vi "IsOpenInterface.vi"(10 "interface handle":i64, 11 "error in (no error)":errorcluster) -> (2 "return type":i8, 3 "error out":errorcluster)   [LabVIEW 2016]
uses:
  MVSDKmd.dll
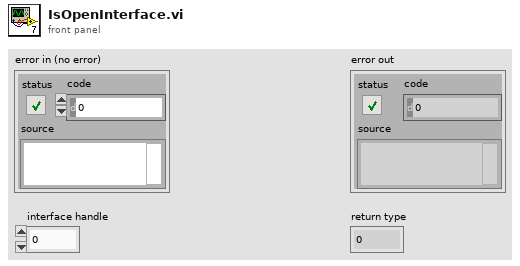
[diagram p1: front panel]
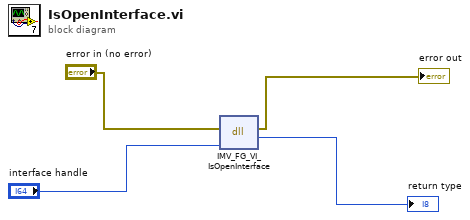
[diagram p0: block diagram]
diagram:
  n1 = dll-call lib="MVSDKmd.dll" fn="IMV_FG_VI_IsOpenInterface"(error in="error in (no error)", "interface handle"="interface handle") -> (error out=→"error out":errorcluster, "return type"=→"return type":i8)  [unwired: 3 in, 1 out]
